vi "Write XBOX USB.vi"(8 "error in (no error)":errorcluster, 10 "JoystickDevice":T1, 11 "Comp Driver in":refnum<class "Comp Driver.lvclass">) -> (0 "error out":errorcluster, 3 "Comp Driver out":refnum<class "Comp Driver.lvclass">)   [LabVIEW 2014, in "Comp Driver.lvlib" / "Comp Driver.lvclass"]
uses:
  Comp Driver.lvclass
  <vilib>/Rock Robotics/WPI/Joystick/WPI_JoystickDeviceEnum.ctl
  Comp Driver.lvclass/Comp Driver.ctl
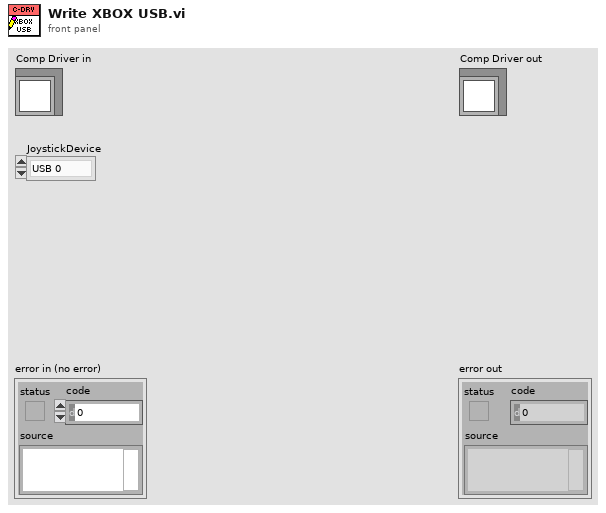
[diagram p1: front panel]
types:
  T1 = typedef "WPI_JoystickDeviceEnum.ctl" = enum16{"USB 0", "USB 1", "USB 2", "USB 3", "USB 4", "USB 5"}
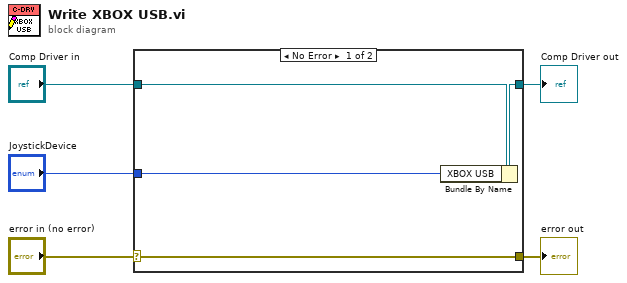
[diagram p0: block diagram]
diagram:
  n1 = case shown="No Error" "error in (no error)" {
    selector: "error in (no error)" -> [w9 w10]
    tunnel: [w9 w10] -> w4
    tunnel: [w7 w11] -> w2
    tunnel: "Comp Driver in" -> [w8 w11]
    tunnel: "JoystickDevice" -> [w6 _]
    frame No Error {
      n2 = Bundle By Name(cluster=w8, "XBOX USB"=w6) -> (w7:refnum<class "Comp Driver.lvclass">)
    }
    frame Error {
    }
  }
  "error out" <- w4
  "Comp Driver out" <- w2
